vi "LWXPS_Example_ReferencingSenserListGet.vi"() -> ()   [LabVIEW 2013]
panel:
  out "Error out":errorcluster caption="error out"
  out "Error code":i32
  out "List":string
  in  "Instrument Key IN":string
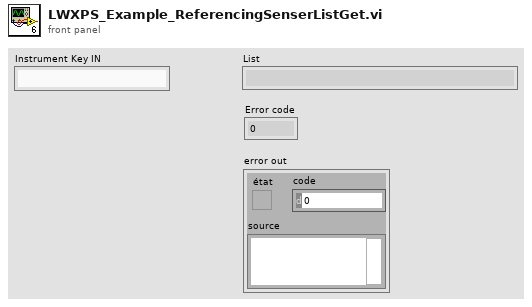
[diagram p1: front panel]
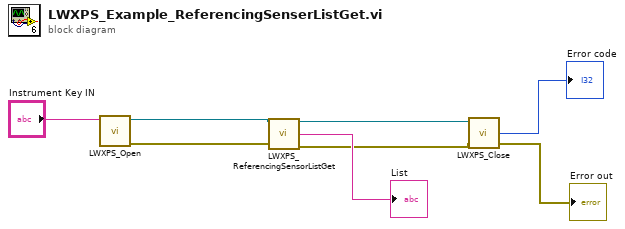
[diagram p0: block diagram]
diagram:
  n1 = call "LWXPS_Open.vi"("Instrument Key IN"="Instrument Key IN") -> ("error out"=w7:errorcluster, "CommandInterfaceXPS.XPS"=w8:refnum<k24>)  [unwired: 3 in, 2 out]
  n2 = call "LWXPS_ReferencingSensorListGet.vi"("XPS Reference IN"=w8, "LabVIEW error IN"=w7) -> ("CommandInterfaceXPS.XPS"=w4:refnum<k24>, "List"=→"List":string, "LabVIEW error OUT"=w3:errorcluster)  [unwired: 9 in, 2 out]
  n3 = call "LWXPS_Close.vi"("error in (no error)"=w3, "XPS Reference"=w4) -> ("Error out"=→"Error out":errorcluster, "Error code"=→"Error code":i32)  [unwired: 2 in]
